vi "Functional Global Variable.vi"(8 "error in":errorcluster, 10 "Operation":T2={"Action"="Modify", "ON(T)OFF(F)"=TRUE, "Func"=enum."Init"}) -> (0 "error out":errorcluster, 1 "ON(T)OFF(F) Out":bool, 2 "Func Out":T1(ring))   [LabVIEW 2017]
doc: "This VI is a Functional Global Variable that will take an initial value from the user, store it in the shift register, increment it then display the result in an indicator"
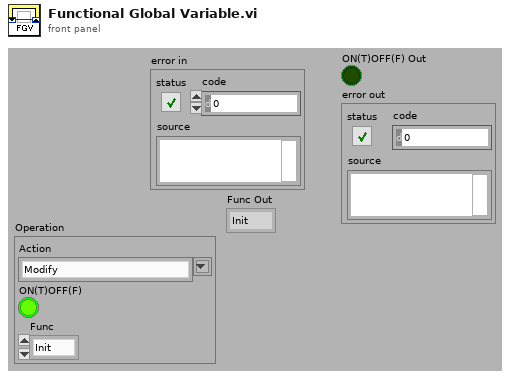
[diagram p1: front panel]
types:
  T1 = enum16{"Init", "VEnable", "PowerOnOff", "PowerONVEnable"}
  T2 = cluster{"Action":string, "ON(T)OFF(F)":bool, "Func":enum16{"Init", "VEnable", "PowerOnOff", "PowerONVEnable"}}
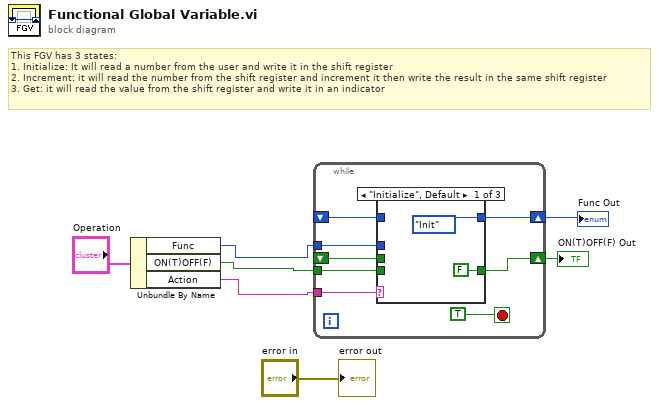
[diagram p0: block diagram]
diagram:
  # "This FGV has 3 states:\n1. Initialize: It will read a number from the user and write it in the shift register\n2. Increment: it will read the number from the shift register and increment it then write the result in the same shift register\n3. Get: it will read the value from the shift register and write it in an indicator"
  n1 = Unbundle By Name("Operation") -> ("Func"=w4:T1, "ON(T)OFF(F)"=w3:bool, "Action"=w2:string)
  n2 = while {
    shift-right: [w15] -> w1
    shift-left: _ -> [w14]
    tunnel: w4 -> [w12]
    tunnel: w3 -> [w11]
    shift-right: [w10] -> w7
    shift-left: _ -> [w9]
    tunnel: w2 -> [w8]
    stop <- TRUE ("stop") stop-if-true
    n3 = case shown="\"Initialize\", Default" w8 {
      tunnel: [T1."Init" ("Func 2") w19 w21] -> w15
      tunnel: w14 -> [_ w19 _]
      tunnel: w12 -> [_ _ w21]
      tunnel: w11 -> [_ _ w20]
      tunnel: [FALSE ("ON(T)OFF(F)") w18 w20] -> w10
      tunnel: w9 -> [_ w18 _]
      frame "Initialize", Default {
      }
      frame "Get" {
      }
      frame "Modify" {
      }
    }
  }
  "ON(T)OFF(F) Out" <- w7
  "Func Out" <- w1
  "error out" <- "error in"
